vi "String Name.vi"() -> (4 "Postfix":string="niDCPower")   [LabVIEW 2021, in "Migrator Reusables.lvlib"]
uses:
  Migrator Reusables.lvlib
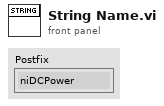
[diagram p1: front panel]
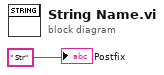
[diagram p0: block diagram]
diagram:
  "Postfix" <- " Str" ("Pin Name")
